vi "MAIN PROGRAM.vi"() -> ()   [LabVIEW 2011]
uses:
  NCML-PhaseSpace/ctrOWLMarker.ctl
  ctlTrialState.ctl
  ctlProtocol.ctl
  ctlProtocolSubID.ctl
  ctlProtocolUnit.ctl
  ctlSeqFNs.ctl
  ctlPkgMain.ctl
  ctlSeqFNs_SubVI PhaseSpace.ctl
  ctlSeqFNs_SubVI ATI.ctl
  ctldistance2plane.ctl
  ctlRecording.ctl
  <vilib>/DAQmx/write.llb/DAQmx Write (Digital 1D U8 1Chan NSamp).vi
  GLOBAL -MAIN.vi
  <vilib>/Utility/file.llb/Write To Spreadsheet File (string).vi
  <vilib>/DAQmx/miscellaneous.llb/DAQmx Fill In Error Info.vi
  <vilib>/Analysis/baseanly.llb/Real Dot Product.vi
  <vilib>/Analysis/NI_AALBase.lvlib
  <vilib>/Utility/VariantDataType/VariantType.lvlib
panel:
  in  "RepeatTrial":bool
  out "Unit Trial count":i32[](array[numeric])
  in  "Recording?":bool=TRUE
  in  "hold criterion (mm)":dbl=250.0 min=0.0 max=500.0 step=1.0
  out "total trials":i32
  in  "Path":path=path "Z:/Yen/NCML-EEGrasp/Data"
  in  "Bias":bool
  out "d (mm)":dbl
  out "ATI":cluster{dbl[][]}[](array[cluster]) {"?" format="%#.2f"}
  out "Current Protocol":T1
  in  "Protocol":T1={"Subject ID"=enum."S000", "1st Handle Left?"=FALSE, "Trial #"=0, "unit"=enum."IL", "unit #"=0, "Trial list"=[], "count in unit"=0, "IL count"=19, "PT count"=3, "postL sessions"=19, "TR max count"=1} {"TR max count" min=1 max=3 step=1; "postL sessions" min=1 max=100 step=1; "PT count" min=1 max=3 step=1}
  out "state":T4
  out "Markers":T5[](array[typedef])
  in  "STOP":bool
  in  "Ready":bool
  out "Date & Time":timestamp format="%<%.3X %x>T"
  # "Main Program"
  # "Recieves data from both SubVIs"
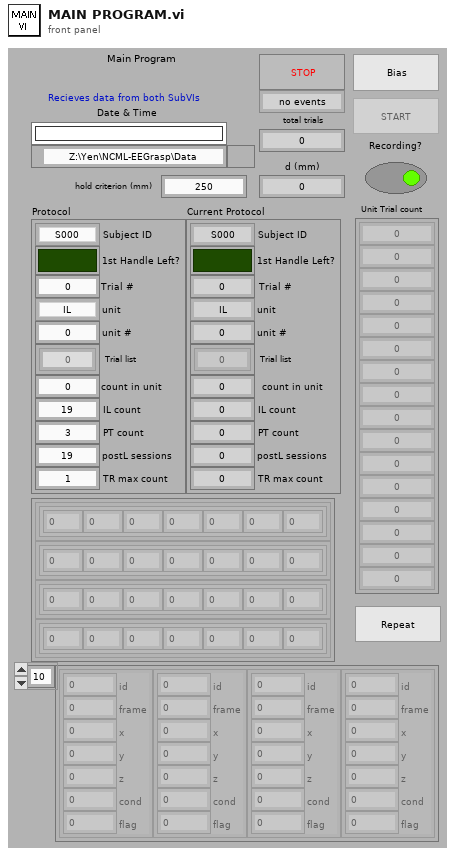
[diagram p1: front panel]
types:
  T1 = typedef "ctlProtocol.ctl" = cluster{"Subject ID":T2, "1st Handle Left?":bool, "Trial #":i32, "unit":T3, "unit #":i32, "Trial list":i32[], "count in unit":i32, "IL count":i32, "PT count":i32, "postL sessions":i32, "TR max count":i32}
  T2 = typedef "ctlProtocolSubID.ctl" = enum16{"S000", "S001", "S002", "S003", "S004", "S005", "S006", "S007"}
  T3 = typedef "ctlProtocolUnit.ctl" = enum16{"IL", "TR", "PT"}
  T4 = typedef "ctlTrialState.ctl" = enum16{"no events", "ready", "start", "hold", "stop", "end"}
  T5 = typedef "ctrOWLMarker.ctl" = cluster{"id":i32, "frame":i32, "x":sgl, "y":sgl, "z":sgl, "cond":sgl, "flag":u32}
  T6 = typedef "ctlPkgMain.ctl" = cluster{"VIRefNm ":refnum<vi>, "PhaseSpace":refnum<queue>, "ATI":refnum<queue>, "Handle Height":dbl, "Results":cluster{"Kc":string, "Cfg":dbl[]}, "CurrPath":path, "state":T4, "tick ini":i64, "Protocol":T1, "PhaseSpace end?":bool, "ATI end?":bool, "trigger task":refnum<k21>, "Markers":T5[], "ATI Data":cluster{dbl[][]}[], "d2plane":T7, "data Path":path, "CurrentProtocol":T1, "tdms data":refnum<k34>, "Recording?":bool}
  T7 = typedef "ctldistance2plane.ctl" = cluster{"1/sqrt(A2+B2+C2)":dbl, "D":dbl, "N":dbl[]}
  T8 = typedef "ctlSeqFNs.ctl" = enum16{"INITIALIZE MAIN", "UpdateProtocol", "UpdatePath", "INITIALIZE Sub", "IDLE", "Bias", "Ready", "RepeatTrial", "Events", "Get PS bias", "Get PhaseSpace", "Get ATI", "Finish", "End PhaseSpace", "End ATI", "ERROR", "EXIT"}
  T9 = enum8{"Enabled", "Disabled", "Disabled and Grayed Out"}
  T10 = typedef "ctlDistance2plane.ctl" = cluster{"1/sqrt(A2+B2+C2)":dbl, "D":dbl, "N":dbl[]}
  T11 = enum16{"ALIGN -CENTER", "ALIGN -TOP LEFT", "ALIGN -AS IS", "ALIGN -CUSTOM"}
  T12 = typedef "ctlSeqFNs_SubVI ATI.ctl" = enum16{"INITIALIZE", "SET HANDLE", "IDLE", "READY", "SEND2MAIN", "CALIB Load", "BIAS", "TRIGGER", "END", "ERROR", "EXIT"}
  T13 = typedef "ctlSeqFNs_SubVI PhaseSpace.ctl" = enum16{"INITIALIZE", "IDLE", "BIAS", "READY", "SEND2MAIN", "LOG2TDMS", "TRIGGER", "END", "ERROR", "EXIT"}
  T14 = enum16{"open", "open or create", "create or replace", "create", "open (read-only)"}
  T15 = typedef "ctlRecording.ctl" = cluster{"recording?":bool, "tdms file":refnum<k34>}
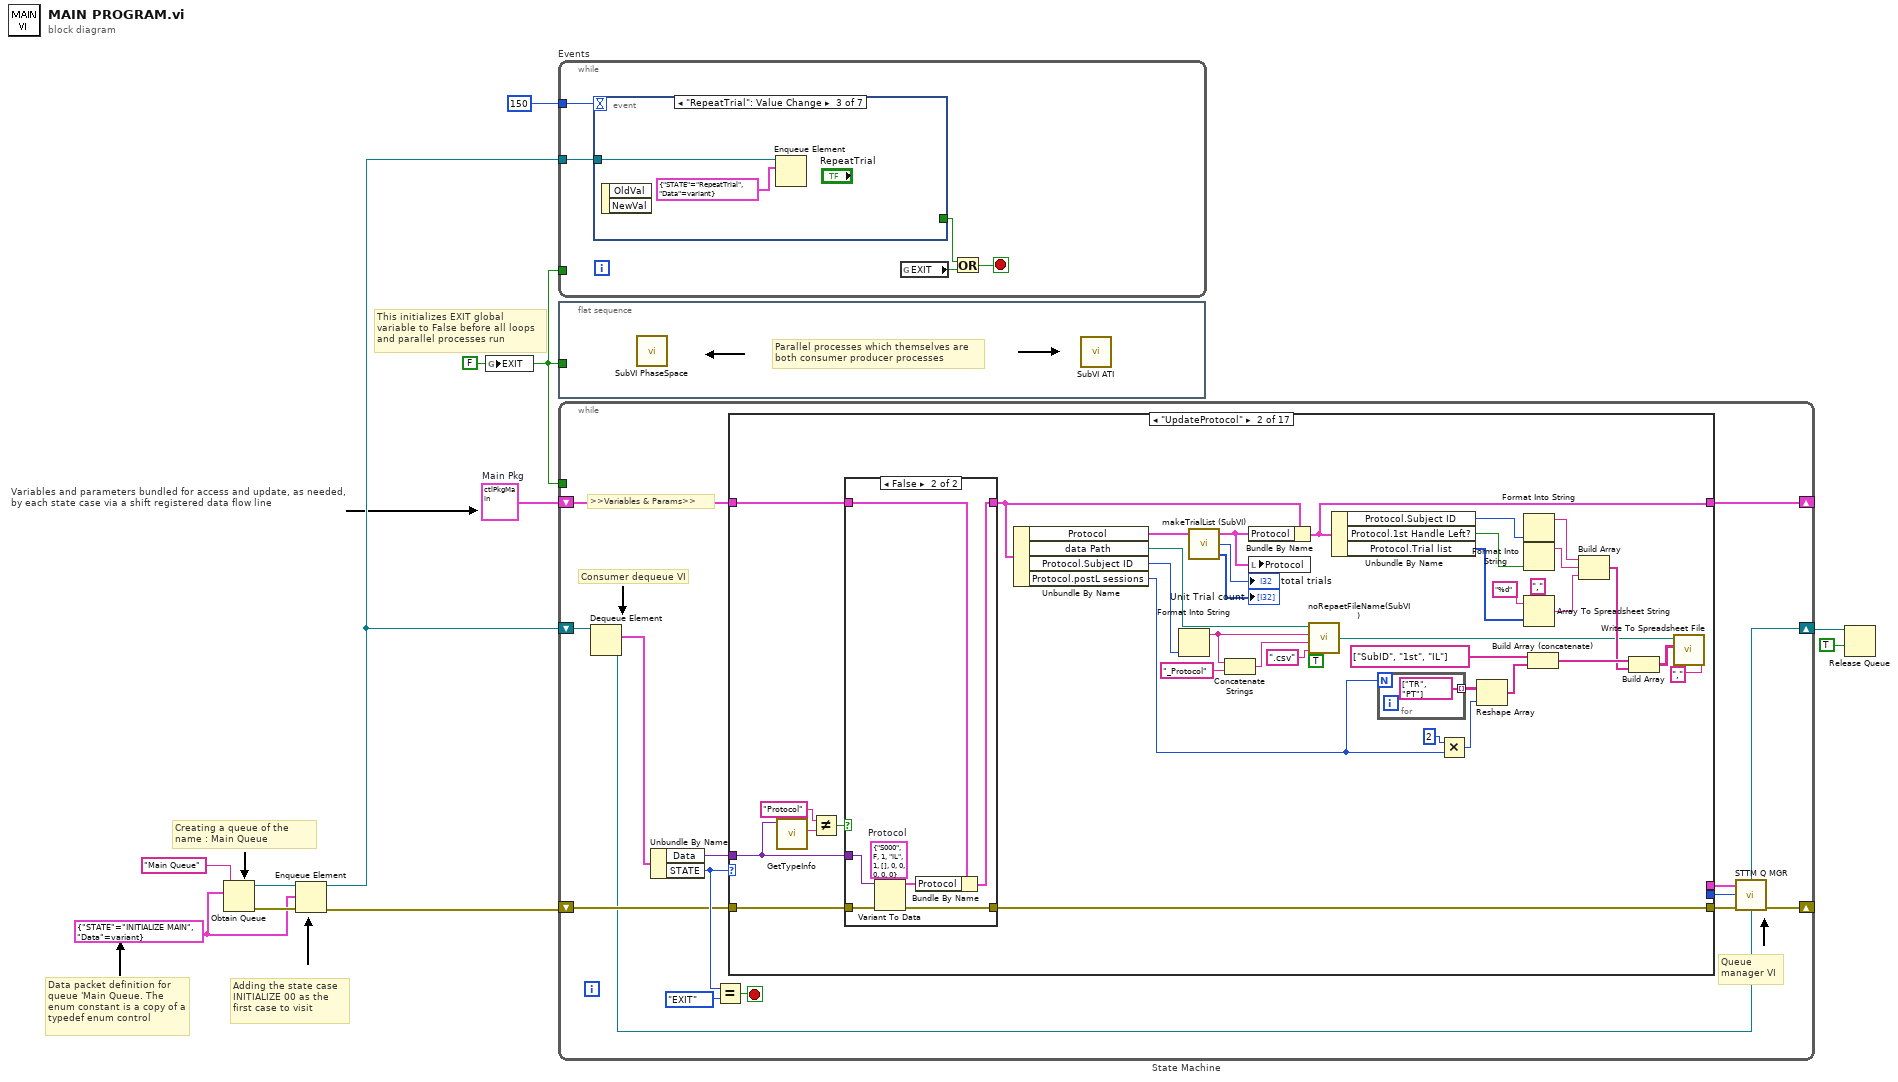
[diagram p0: block diagram]
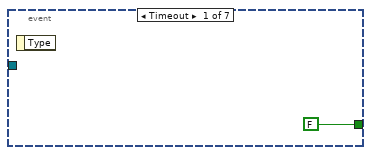
[diagram p2: hidden frame]
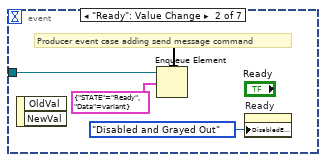
[diagram p3: hidden frame]
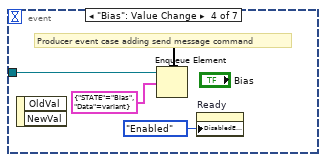
[diagram p4: hidden frame]
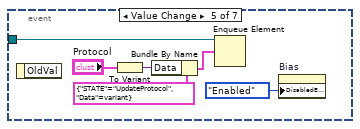
[diagram p5: hidden frame]
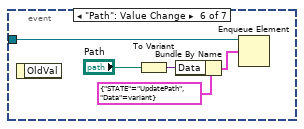
[diagram p6: hidden frame]
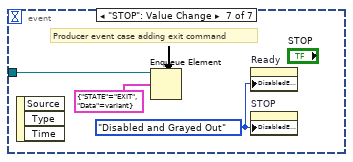
[diagram p7: hidden frame]
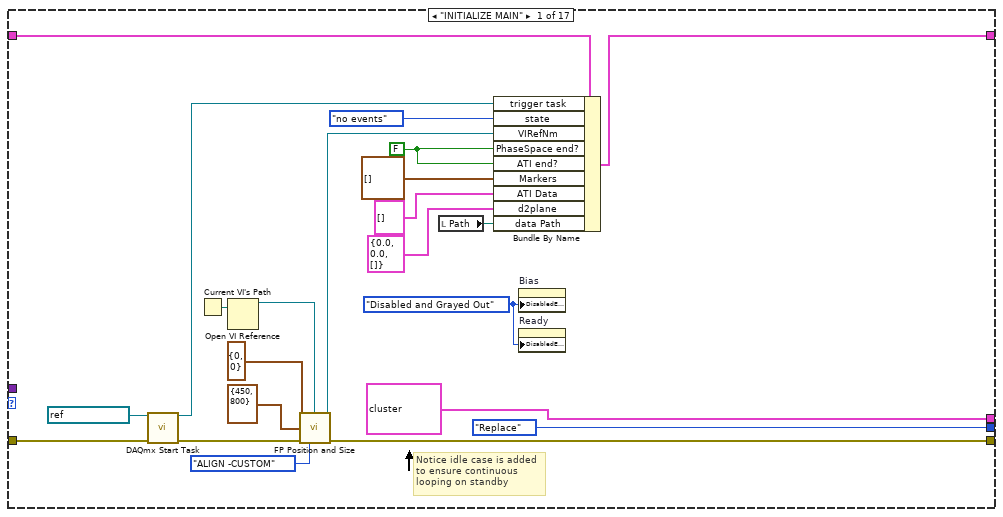
[diagram p8: hidden frame]
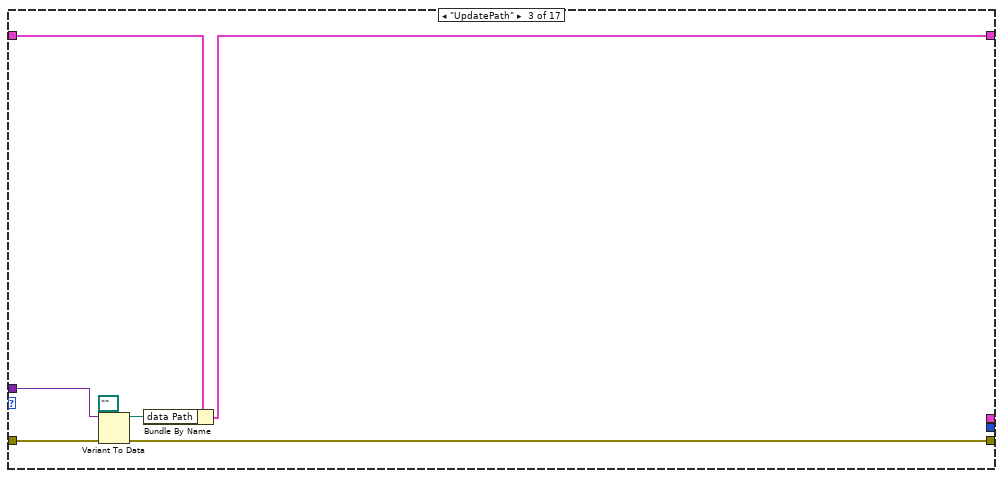
[diagram p10: hidden frame]
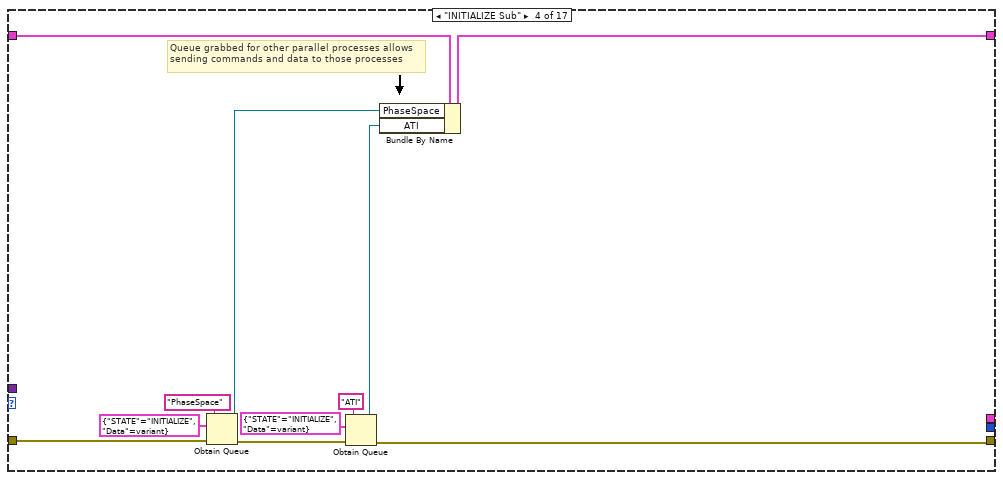
[diagram p11: hidden frame]
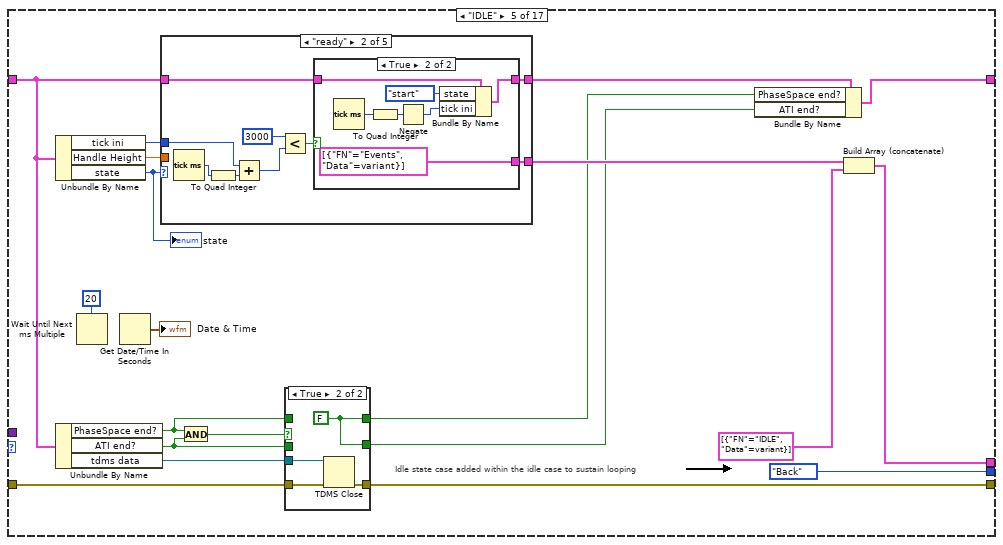
[diagram p12: hidden frame]
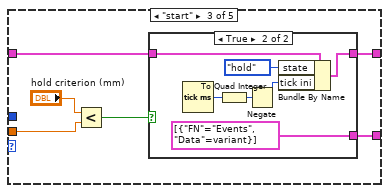
[diagram p16: hidden frame]
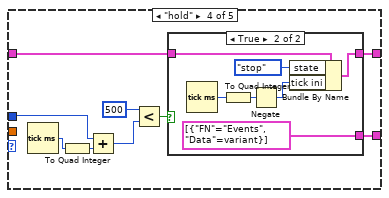
[diagram p18: hidden frame]
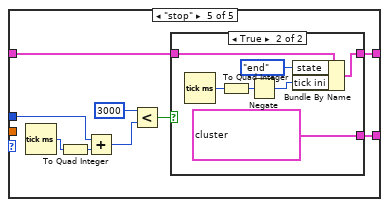
[diagram p20: hidden frame]
diagram:
  w1 = T6 {"VIRefNm "=refnum, "PhaseSpace"=refnum, "ATI"=refnum, "Handle Height"=0.0, "Results"={"Kc"="", "Cfg"=[]}, "CurrPath"=path "", "state"=enum."no events", "tick ini"=0, "Protocol"={"Subject ID"=enum."S000", "1st Handle Left?"=FALSE, "Trial #"=0, "unit"=enum."IL", "unit #"=0, "Trial list"=[], "count in unit"=0, "IL count"=0, "PT count"=0, "postL sessions"=0, "TR max count"=0}, "PhaseSpace end?"=FALSE, "ATI end?"=FALSE, "trigger task"="", "Markers"=[], "ATI Data"=[], "d2plane"={"1/sqrt(A2+B2+C2)"=0.0, "D"=0.0, "N"=[]}, "data Path"=path "", "CurrentProtocol"={"Subject ID"=enum."S000", "1st Handle Left?"=FALSE, "Trial #"=0, "unit"=enum."IL", "unit #"=0, "Trial list"=[], "count in unit"=0, "IL count"=0, "PT count"=0, "postL sessions"=0, "TR max count"=0}, "tdms data"=refnum, "Recording?"=FALSE}  # Main Pkg
  w4 = FALSE
  w5 = cluster{"STATE":T8, "Data":variant} {"STATE"=enum."INITIALIZE MAIN", "Data"=variant} ("element")
  # "This initializes EXIT global variable to False before all loops and parallel processes run"
  # "Data packet definition for queue 'Main Queue. The enum constant is a copy of a typedef enum control"
  # "Adding the state case INITIALIZE 00 as the first case to visit"
  # "Creating a queue of the name : Main Queue"
  # "Variables and parameters bundled for access and update, as needed,  by each state case via a shift registered data flow line"
  n1 = Obtain Queue(name (unnamed)="Main Queue" ("Queue Name"), element data type=w5) -> (queue out=w3:refnum<queue>, error out=w7:errorcluster)  [unwired: 3 in, 1 out]
  n2 = Enqueue Element(queue=w3, element=w5, error in (no error)=w7) -> (queue out=w2:refnum<queue>, error out=w6:errorcluster)  [unwired: 1 in, 1 out]
  n3 = global write "GLOBAL -MAIN.vi" "EXIT"(w4) -> ()
  n4 = while "Events" {
    tunnel: 150 -> [w16]
    tunnel: w4 -> [_]
    tunnel: w2 -> [w12]
    stop <- w13 stop-if-true
    n5 = event shown="[2] \"RepeatTrial\": Value Change" {
      selector: _ -> [_ _ _ _ _ _ _]
      dyn-events: _ -> [_ _ _ _ _ _ _]
      timeout: w16 -> [_ _ _ _ _ _ _]
      tunnel: [FALSE _ _ _ _ _ _] -> w15
      tunnel: w12 -> [_ w20 w22 w25 w30 w35 w39]
      event Timeout {
        n6 = event-data() -> ()  [unwired: 1 in, 1 out]
      }
      event "Ready": Value Change {
        # "Producer event case adding send message command"
        n7 = event-data() -> ()  [unwired: 1 in, 2 out]
        n8 = Enqueue Element(queue=w20, element=cluster{"STATE":T8, "Data":variant} {"STATE"=enum."Ready", "Data"=variant}) -> ()  [unwired: 2 in, 3 out]
        n9 = property on="Ready" class="Bool"("DisabledEnum"=T9."Disabled and Grayed Out" ("Disabled")) -> ()  [unwired: 2 in, 2 out]
      }
      event "RepeatTrial": Value Change {
        n10 = event-data() -> ()  [unwired: 1 in, 2 out]
        n11 = Enqueue Element(queue=w22, element=cluster{"STATE":T8, "Data":variant} {"STATE"=enum."RepeatTrial", "Data"=variant}) -> ()  [unwired: 2 in, 3 out]
      }
      event "Bias": Value Change {
        # "Producer event case adding send message command"
        n12 = event-data() -> ()  [unwired: 1 in, 2 out]
        n13 = Enqueue Element(queue=w25, element=cluster{"STATE":T8, "Data":variant} {"STATE"=enum."Bias", "Data"=variant}) -> ()  [unwired: 2 in, 3 out]
        n14 = property on="Ready" class="Bool"("DisabledEnum"=T9."Enabled" ("Disabled")) -> ()  [unwired: 2 in, 2 out]
      }
      event Value Change {
        n15 = event-data() -> ()  [unwired: 1 in, 1 out]
        n16 = To Variant(anything="Protocol") -> (Variant=w28:variant)
        n17 = Bundle By Name(cluster=cluster{"STATE":T8, "Data":variant} {"STATE"=enum."UpdateProtocol", "Data"=variant} ("element"), "Data"=w28) -> (w29:cluster{"STATE":T8, "Data":variant})
        n18 = Enqueue Element(queue=w30, element=w29) -> ()  [unwired: 2 in, 3 out]
        n19 = property on="Bias" class="Bool"("DisabledEnum"=T9."Enabled" ("Disabled")) -> ()  [unwired: 2 in, 2 out]
      }
      event "Path": Value Change {
        n20 = event-data() -> ()  [unwired: 1 in, 1 out]
        n21 = To Variant(anything="Path") -> (Variant=w33:variant)
        n22 = Bundle By Name(cluster=cluster{"STATE":T8, "Data":variant} {"STATE"=enum."UpdatePath", "Data"=variant} ("element"), "Data"=w33) -> (w34:cluster{"STATE":T8, "Data":variant})
        n23 = Enqueue Element(queue=w35, element=w34) -> ()  [unwired: 2 in, 3 out]
      }
      event "STOP": Value Change {
        w37 = T9."Disabled and Grayed Out" ("Disabled")
        # "Producer event case adding exit command"
        n24 = event-data() -> ()  [unwired: 1 in, 3 out]
        n25 = Enqueue Element(queue=w39, element=cluster{"STATE":T8, "Data":variant} {"STATE"=enum."EXIT", "Data"=variant}) -> ()  [unwired: 2 in, 3 out]
        n26 = property on="Ready" class="Bool"("DisabledEnum"=w37) -> ()  [unwired: 2 in, 2 out]
        n27 = property on="STOP" class="Bool"("DisabledEnum"=w37) -> ()  [unwired: 2 in, 2 out]
      }
    }
    n28 = global read "GLOBAL -MAIN.vi" "EXIT"() -> (w14:bool)
    n29 = Or(x=w15, y=w14) -> (x .or. y?=w13:bool)
  }
  n30 = flat-sequence {
    tunnel: w4 -> [_]
    frame #0 {
      # "Parallel processes which themselves are both consumer producer processes"
      n31 = call "SubVI PhaseSpace.vi"() -> ()  [unwired: 16 in]
      n32 = call "SubVI ATI.vi"() -> ()  [unwired: 16 in]
    }
  }
  n33 = while "State Machine" {
    shift-right: [w47] -> _
    shift-left: w6 -> [w46]
    shift-right: [w40] -> w9
    shift-left: w2 -> [w53]
    tunnel: w4 -> [_]
    shift-right: [w43] -> _
    shift-left: w1 -> [w44]
    stop <- w45 stop-if-true
    # "Queue manager VI"
    # "Consumer dequeue VI"
    # ">>Variables & Params>>"
    n34 = Dequeue Element(queue=w53) -> (queue out=w40:refnum<queue>, element=w52:cluster{"STATE":T8, "Data":variant})  [unwired: 2 in, 2 out]
    n35 = Unbundle By Name(w52) -> ("Data"=w51:variant, "STATE"=w50:T8)
    n36 = Equal?(x=w50, y=ctlSeqFNs."EXIT" ("FN")) -> (x = y?=w45:bool)
    n37 = case shown="\"UpdateProtocol\"" w50 {
      tunnel: w46 -> [w60 w112 w128 w132 w151 w243 w277 w287 w305 w363 w371 w378 w398 w400 w404 w408 w411]
      tunnel: [w70 w113 w129 w133 w150 w241 w274 w287 w300 w362 w370 w377 w391 w400 w404 w407 w414] -> w48
      tunnel: w51 -> [_ w111 w127 _ _ _ _ _ _ w365 w372 w379 _ _ _ _ _]
      tunnel: [cluster{"FN":T8, "Data":variant}[] [{"FN"=enum."INITIALIZE Sub", "Data"=variant}, {"FN"=enum."IDLE", "Data"=variant}] _ _ _ w157 _ cluster{"FN":T8, "Data":variant}[] [{"FN"=enum."Events", "Data"=variant}] _ _ _ _ _ _ _ _ _ _] -> w41
      tunnel: w44 -> [w64 w114 w131 w142 w152 w237 w259 w285 w314 w349 w369 w375 w380 w402 w406 w409 w420]
      tunnel: [w69 w86 w130 w141 w148 w237 w275 w286 w314 w361 w368 w374 w381 w401 w405 w409 w420] -> w43
      tunnel: [enum16{"Back", "Front", "Replace"}."Replace" ("FNs") _ _ _ enum16{"Back", "Front", "Replace"}."Back" ("FNs") _ enum16{"Back", "Front", "Replace"}."Front" ("FNs") _ _ _ _ _ _ _ _ _ _] -> w42
      frame "INITIALIZE MAIN" {
        w54 = T9."Disabled and Grayed Out" ("Disabled")
        w63 = FALSE ("PhaseSpace end?")
        # "Notice idle case is added to ensure continuous looping on standby"
        n38 = call <vilib>:"DAQmx Start Task.vi"("task/channels in"=refnum<k21> "TriggerPort" ("DAQmx Task Name"), "error in"=w60) -> ("task out"=w61:refnum<k21>, "error out"=w59:errorcluster)  [unwired: 12 in]
        n39 = Current VI's Path() -> (path=w71:path)
        n40 = Open VI Reference(vi path=w71) -> (vi reference=w72:refnum<vi>)  [unwired: 5 in, 1 out]
        n41 = call "FP Position and Size.vi"("VIRefNum  IN"=w72, "Poistion"=cluster{"left":i16, "top":i16} {"left"=0, "top"=0}, "Size"=cluster{"right":i16, "bottom":i16} {"right"=450, "bottom"=800}, "error in (no error)"=w59, "Mode"=T11."ALIGN -CUSTOM") -> ("VIRefNum OUT"=w68:refnum<vi>, "error out"=w70:errorcluster)  [unwired: 9 in]
        n42 = local read "Path"() -> (w55:path)
        n43 = Bundle By Name(cluster=w64, "trigger task"=w61, "state"=ctlTrialState."no events", "VIRefNm"=w68, "PhaseSpace end?"=w63, "ATI end?"=w63, "Markers"=T5[] [], "ATI Data"=cluster{dbl[][]}[] [] ("Data"), "d2plane"=T10 {"1/sqrt(A2+B2+C2)"=0.0, "D"=0.0, "N"=[]}, "data Path"=w55) -> (w69:T6)
        n44 = property on="Bias" class="Bool"("DisabledEnum"=w54) -> ()  [unwired: 2 in, 2 out]
        n45 = property on="Ready" class="Bool"("DisabledEnum"=w54) -> ()  [unwired: 2 in, 2 out]
      }
      frame "UpdateProtocol" {
        n46 = call <vilib>:"GetTypeInfo.vi"("Variant"=w111) -> ("Name"=w110:string)  [unwired: 6 in, 4 out]
        n47 = Not Equal?(x="Protocol", y=w110) -> (x != y?=w108:bool)
        n48 = case shown="False" w108 {
          tunnel: w114 -> [w117 w124]
          tunnel: [w117 w123] -> w88
          tunnel: [w116 w118] -> w113
          tunnel: w112 -> [w116 w120]
          tunnel: w111 -> [_ w119]
          frame True {
          }
          frame False {
            w122 = T1 {"Subject ID"=enum."S000", "1st Handle Left?"=FALSE, "Trial #"=1, "unit"=enum."IL", "unit #"=1, "Trial list"=[], "count in unit"=0, "IL count"=0, "PT count"=0, "postL sessions"=0, "TR max count"=0}  # Protocol
            n49 = Variant To Data(error in=w120, type=w122, Variant=w119) -> (data=w121:T1, error out=w118:errorcluster)
            n50 = Bundle By Name(cluster=w124, "Protocol"=w121) -> (w123:T6)
          }
        }
        n51 = Unbundle By Name(w88) -> ("Protocol"=w89:T1, "data Path"=w81:path, "Protocol.Subject ID"=w82:T2, "Protocol.postL sessions"=w83:i32)
        n52 = Format Into String(w82) -> (resulting string=w80:string)  [unwired: 3 in, 1 out]
        n53 = call "makeTrialList (SubVI).vi"("Protocol in"=w89) -> ("Unit Trial count"=→"Unit Trial count":i32[], "total trial count"=→"total trials":i32, "Protocol out"=w87:T1)  [unwired: 2 in]
        n54 = Concatenate Strings(w80, "_Protocol") -> (w79:string)
        n55 = Bundle By Name(cluster=w88, "Protocol"=w87) -> (w86:T6)
        n56 = local write "Protocol"(w87) -> ()
        n57 = call "noRepaetFileName(SubVI).vi"("prompt overwrite?"=TRUE, "ext"=".csv" ("string"), "file name"=w79, "subID"=w80, "directory Path"=w81) -> ("file path out"=w76:path)  [unwired: 1 in]
        n58 = Unbundle By Name(w86) -> ("Protocol.Subject ID"=w100:T2, "Protocol.1st Handle Left?"=w99:bool, "Protocol.Trial list"=w96:i32[])
        n59 = for {
          N: w83 -> [_]
          tunnel: [string[] ["TR", "PT"]] -> w106 mode=indexing
        }
        n60 = Multiply(x=2 ("y"), y=w83) -> (x*y=w105:i32)
        n61 = Reshape Array(w106, w105) -> (w104:string[])
        n62 = Format Into String(w100) -> (resulting string=w98:string)  [unwired: 3 in, 1 out]
        n63 = Format Into String(w99) -> (resulting string=w97:string)  [unwired: 3 in, 1 out]
        n64 = Array To Spreadsheet String(delimiter (Tab)=",", array=w96, 3:"%d" ("format string")) -> (spreadsheet string=w94:string)
        n65 = Build Array (concatenate)(string[] ["SubID", "1st", "IL"], w104) -> (w102:string[])
        n66 = Build Array(w98, w97, w94) -> (w92:string[])
        n67 = Build Array(w102, w92) -> (w93:string[][])
        n68 = call-poly <vilib>:"Write To Spreadsheet File.vi"("delimiter (\\t)"="," ("delimiter (\\t)"), "2D data"=w93, "file path (dialog if empty)"=w76) -> ()  [unwired: 5 in, 1 out]
      }
      frame "UpdatePath" {
        n69 = Variant To Data(error in=w128, type=path "", Variant=w127) -> (data=w126:path, error out=w129:errorcluster)
        n70 = Bundle By Name(cluster=w131, "data Path"=w126) -> (w130:T6)
      }
      frame "INITIALIZE Sub" {
        # "Queue grabbed for other parallel processes allows sending commands and data to those processes"
        n71 = Obtain Queue(name (unnamed)="PhaseSpace", element data type=cluster{"STATE":T13, "Data":variant} {"STATE"=enum."INITIALIZE", "Data"=variant} ("element"), error in (no error)=w132) -> (queue out=w135:refnum<queue>, error out=w140:errorcluster)  [unwired: 2 in, 1 out]
        n72 = Obtain Queue(name (unnamed)="ATI", element data type=cluster{"STATE":T12, "Data":variant} {"STATE"=enum."INITIALIZE", "Data"=variant} ("element"), error in (no error)=w140) -> (queue out=w134:refnum<queue>, error out=w133:errorcluster)  [unwired: 2 in, 1 out]
        n73 = Bundle By Name(cluster=w142, "PhaseSpace"=w135, "ATI"=w134) -> (w141:T6)
      }
      frame "IDLE" {
        # "Idle state case added within the idle case to sustain looping"
        n74 = Unbundle By Name(w152) -> ("tick ini"=w154:i64, "Handle Height"=w159:dbl, "state"=w160:T4)
        "state" <- w160
        n75 = Unbundle By Name(w152) -> ("PhaseSpace end?"=w144:bool, "ATI end?"=w147:bool, "tdms data"=w153:refnum<k34>)
        n76 = Wait Until Next ms Multiple(millisecond multiple=u32 20) -> ()  [unwired: 1 out]
        n77 = Get Date/Time In Seconds() -> (seconds since 1Jan1904=→"Date & Time":timestamp)
        n78 = case shown="\"ready\"" w160 {
          tunnel: w159 -> [_ _ w189 _ _]
          tunnel: w152 -> [w170 w179 w193 w210 w227]
          tunnel: [w170 w178 w192 w209 w226] -> w149
          tunnel: [_ w177 w188 w208 w225] -> w155
          tunnel: w154 -> [_ w175 _ w203 w220]
          frame "no events", Default {
          }
          frame "ready" {
            n79 = Tick Count (ms)() -> (millisecond timer value=w176:u32)
            n80 = To Quad Integer(1:w176) -> (0:w174:i64)
            n81 = Add(x=w175, y=w174) -> (x+y=w172:i64)
            n82 = Less?(x=i64 3000 ("Time Target (s)"), y=w172) -> (x < y?=w173:bool)
            n83 = case shown="True" w173 {
              tunnel: w179 -> [w180 w187]
              tunnel: [w180 w186] -> w178
              tunnel: [_ cluster{"FN":T8, "Data":variant}[] [{"FN"=enum."Events", "Data"=variant}]] -> w177
              frame False {
              }
              frame True {
                n84 = Tick Count (ms)() -> (millisecond timer value=w182:u32)
                n85 = To Quad Integer(1:w182) -> (0:w183:i64)
                n86 = Negate(x=w183) -> (-x=w181:i64)
                n87 = Bundle By Name(cluster=w187, "state"=ctlTrialState."start", "tick ini"=w181) -> (w186:T6)
              }
            }
          }
          frame "start" {
            n88 = Less?(x="hold criterion (mm)", y=w189) -> (x < y?=w191:bool)
            n89 = case shown="True" w191 {
              tunnel: w193 -> [w194 w201]
              tunnel: [w194 w200] -> w192
              tunnel: [_ cluster{"FN":T8, "Data":variant}[] [{"FN"=enum."Events", "Data"=variant}]] -> w188
              frame False {
              }
              frame True {
                n90 = Tick Count (ms)() -> (millisecond timer value=w197:u32)
                n91 = To Quad Integer(1:w197) -> (0:w196:i64)
                n92 = Negate(x=w196) -> (-x=w195:i64)
                n93 = Bundle By Name(cluster=w201, "state"=ctlTrialState."hold", "tick ini"=w195) -> (w200:T6)
              }
            }
          }
          frame "hold" {
            n94 = Tick Count (ms)() -> (millisecond timer value=w207:u32)
            n95 = To Quad Integer(1:w207) -> (0:w206:i64)
            n96 = Add(x=w203, y=w206) -> (x+y=w205:i64)
            n97 = Less?(x=i64 500 ("Time Target (s)"), y=w205) -> (x < y?=w202:bool)
            n98 = case shown="True" w202 {
              tunnel: w210 -> [w211 w218]
              tunnel: [w211 w217] -> w209
              tunnel: [_ cluster{"FN":T8, "Data":variant}[] [{"FN"=enum."Events", "Data"=variant}]] -> w208
              frame False {
              }
              frame True {
                n99 = Tick Count (ms)() -> (millisecond timer value=w214:u32)
                n100 = To Quad Integer(1:w214) -> (0:w213:i64)
                n101 = Negate(x=w213) -> (-x=w212:i64)
                n102 = Bundle By Name(cluster=w218, "state"=ctlTrialState."stop", "tick ini"=w212) -> (w217:T6)
              }
            }
          }
          frame "stop" {
            n103 = Tick Count (ms)() -> (millisecond timer value=w224:u32)
            n104 = To Quad Integer(1:w224) -> (0:w223:i64)
            n105 = Add(x=w220, y=w223) -> (x+y=w222:i64)
            n106 = Less?(x=i64 3000 ("Time Target (s)"), y=w222) -> (x < y?=w219:bool)
            n107 = case shown="True" w219 {
              tunnel: w227 -> [w228 w235]
              tunnel: [w228 w234] -> w226
              tunnel: [_ cluster{"FN":T8, "Data":variant}[] [{"FN"=enum."Events", "Data"=variant}, {"FN"=enum."Finish", "Data"=variant}]] -> w225
              frame False {
              }
              frame True {
                n108 = Tick Count (ms)() -> (millisecond timer value=w230:u32)
                n109 = To Quad Integer(1:w230) -> (0:w231:i64)
                n110 = Negate(x=w231) -> (-x=w229:i64)
                n111 = Bundle By Name(cluster=w235, "state"=ctlTrialState."end", "tick ini"=w229) -> (w234:T6)
              }
            }
          }
        }
        n112 = And(x=w144, y=w147) -> (x .and. y?=w143:bool)
        n113 = case shown="True" w143 {
          tunnel: w153 -> [_ w169]
          tunnel: w151 -> [w165 w168]
          tunnel: [w165 w167] -> w150
          tunnel: [w164 w166] -> w146
          tunnel: w144 -> [w164 _]
          tunnel: [w163 w166] -> w145
          tunnel: w147 -> [w163 _]
          frame False {
          }
          frame True {
            w166 = FALSE
            n114 = TDMS Close(8:w168, 11:w169) -> (0:w167:errorcluster)  [unwired: 1 out]
          }
        }
        n115 = Bundle By Name(cluster=w149, "PhaseSpace end?"=w146, "ATI end?"=w145) -> (w148:T6)
        n116 = Build Array (concatenate)(w155, cluster{"FN":T8, "Data":variant}[] [{"FN"=enum."IDLE", "Data"=variant}]) -> (w157:cluster{"FN":T8, "Data":variant}[])
      }
      frame "Bias" {
        n117 = Unbundle By Name(w237) -> ("PhaseSpace"=w239:refnum<queue>, "ATI"=w240:refnum<queue>)
        n118 = Enqueue Element(queue=w240, element=cluster{"STATE":T12, "Data":variant} {"STATE"=enum."BIAS", "Data"=variant}, error in (no error)=w243) -> (error out=w242:errorcluster)  [unwired: 1 in, 2 out]
        n119 = Enqueue Element(queue=w239, element=cluster{"STATE":T13, "Data":variant} {"STATE"=enum."BIAS", "Data"=variant}, error in (no error)=w242) -> (error out=w241:errorcluster)  [unwired: 1 in, 2 out]
      }
      frame "Ready" {
        n120 = Unbundle By Name(w259) -> ("Protocol"=w245:T1, "data Path"=w256:path, "PhaseSpace"=w263:refnum<queue>, "ATI"=w264:refnum<queue>)
        n121 = in-place {
          n122 = in-place-cluster #1(w245) -> ("Trial #"=w280:i32, "unit #"=w283:i32, "count in unit"=w282:i32)
          n123 = Increment(x=w280) -> (x+1=w278:i32)
          n124 = Increment(x=w282) -> (x+1=w279:i32)
          n125 = Increment(x=w283) -> (x+1=w281:i32)
          n126 = in-place-cluster #1("Trial #"=w278, "unit #"=w281, "count in unit"=w279) -> (→"Current Protocol":T1)
        }
        n127 = call "updateTrialInfo (SubVI).vi"("data Path"=w256, "pre Protocol"=w245) -> ("file path out"=w252:path, "next"=w246:T1)
        n128 = Strip Path(path=w252) -> (stripped path=w251:path)  [unwired: 1 out]
        n129 = Build Path(base path=w251, name or relative path="dummy") -> (appended path=w249:path)
        n130 = Select(t=w252, s="Recording?", f=w249) -> (s? t:f=w253:path)
        n131 = TDMS Open(6:FALSE ("disable buffering? (T)"), 10:T14."create or replace" ("operation"), 11:w253) -> (3:w248:refnum<k34>)  [unwired: 3 in, 1 out]
        n132 = Bundle By Name(cluster=T15 {"recording?"=FALSE, "tdms file"=refnum} ("output cluster"), "tdms file"=w248, "recording?"="Recording?") -> (w257:T15)
        n133 = Tick Count (ms)() -> (millisecond timer value=w267:u32)
        n134 = To Quad Integer(1:w267) -> (0:w266:i64)
        n135 = To Variant(anything=w257) -> (Variant=w262:variant)
        n136 = Negate(x=w266) -> (-x=w265:i64)
        n137 = Bundle By Name(cluster=cluster{"STATE":T12, "Data":variant} {"STATE"=enum."READY", "Data"=variant} ("element"), "Data"=w262) -> (w260:cluster{"STATE":T12, "Data":variant})
        n138 = Bundle By Name(cluster=w259, "CurrentProtocol"=w245, "Protocol"=w246, "state"=ctlTrialState."ready", "tick ini"=w265, "tdms data"=w248, "Recording?"="Recording?") -> (w275:T6)
        n139 = Enqueue Element(queue=w264, element=w260, error in (no error)=w277) -> (error out=w276:errorcluster)  [unwired: 1 in, 2 out]
        n140 = To Variant(anything=w257) -> (Variant=w268:variant)
        n141 = Bundle By Name(cluster=cluster{"STATE":T13, "Data":variant} {"STATE"=enum."READY", "Data"=variant} ("element"), "Data"=w268) -> (w269:cluster{"STATE":T13, "Data":variant})
        n142 = Enqueue Element(queue=w263, element=w269, error in (no error)=w276) -> (error out=w274:errorcluster)  [unwired: 1 in, 2 out]
      }
      frame "RepeatTrial" {
        n143 = Unbundle By Name(w285) -> ("CurrentProtocol"=w284:T1)
        n144 = Bundle By Name(cluster=w285, "Protocol"=w284) -> (w286:T6)
      }
      frame "Events" {
        n145 = Unbundle By Name(w314) -> ("PhaseSpace"=w291:refnum<queue>, "ATI"=w290:refnum<queue>, "CurrentProtocol.unit"=w288:T3, "CurrentProtocol.1st Handle Left?"=w289:bool, "state"=w308:T4, "trigger task"=w307:refnum<k21>)
        n146 = case shown="\"start\"" w308 {
          selector: w308 -> [w321 w324 w335 w338 w341 w344]
          tunnel: [w321 w324 w335 w338 w341 w344] -> w313
          tunnel: [u8 0 ("element") u8 9 ("element") u8 17 ("element") u8 33 ("element") u8 65 ("element") u8 129 ("element")] -> w310
          tunnel: ["Finish" ("name or relative path") "Ready" ("name or relative path") w326 "Hold" ("name or relative path") "Relax" ("name or relative path") "Finish" ("name or relative path")] -> w295
          tunnel: w289 -> [_ _ w325 _ _ _]
          tunnel: w288 -> [_ _ w328 _ _ _]
          frame "no events", Default {
          }
          frame "ready" {
          }
          frame "start" {
            n147 = Not Equal?(x=w328, y=ctlProtocolUnit."TR" ("Protocol.unit")) -> (x != y?=w329:bool)
            n148 = Not(x=w325) -> (.not. x?=w330:bool)
            n149 = Select(t=w325, s=w329, f=w330) -> (s? t:f=w332:bool)
            n150 = Select(t="Left" ("name or relative path"), s=w332, f="RIght") -> (s? t:f=w326:string)
          }
          frame "hold" {
          }
          frame "stop" {
          }
          frame "end" {
          }
        }
        n151 = To Variant(anything=w313) -> (Variant=w312:variant)
        n152 = Build Array(w310, u8 0 ("element")) -> (w311:u8[])
        n153 = Bundle By Name(cluster=cluster{"STATE":T12, "Data":variant} {"STATE"=enum."TRIGGER", "Data"=variant} ("element"), "Data"=w312) -> (w315:cluster{"STATE":T12, "Data":variant})
        n154 = Enqueue Element(queue=w290, element=w315, error in (no error)=w305) -> (error out=w306:errorcluster)  [unwired: 1 in, 2 out]
        n155 = call-poly <vilib>:"DAQmx Write.vi"("task/channels in"=w307, "data"=w311, "error in"=w305) -> ("error out"=w303:errorcluster)  [unwired: 10 in, 2 out]
        n156 = Bundle By Name(cluster=cluster{"STATE":T13, "Data":variant} {"STATE"=enum."TRIGGER", "Data"=variant} ("element"), "Data"=w312) -> (w316:cluster{"STATE":T13, "Data":variant})
        n157 = Enqueue Element(queue=w291, element=w316, error in (no error)=w305) -> (error out=w304:errorcluster)  [unwired: 1 in, 2 out]
        n158 = call <vilib>:"Application Directory.vi"() -> ("Application Directory"=w297:path)
        n159 = Merge Errors(w304, w306, w303) -> (w299:errorcluster)
        n160 = Build Path(base path=w297, name or relative path="audio cues") -> (appended path=w294:path)
        n161 = Concatenate Strings(w295, ".wav" ("name or relative path")) -> (w293:string)
        n162 = Build Path(base path=w294, name or relative path=w293) -> (appended path=w292:path)
        n163 = call <vilib>:"Sound File Read Simple.vi"("error in (no error)"=w299, "path"=w292) -> ("error out"=w301:errorcluster, "data"=w302:waveform(dbl)[])  [unwired: 6 in, 2 out]
        n164 = call "Play Waveform"("Data"=w302, "error in"=w301) -> ("error out"=w300:errorcluster)  [unwired: 17 in]
      }
      frame "Get PhaseSpace" {
        n165 = Variant To Data(error in=w363, type=T5[] [] ("Markers"), Variant=w365) -> (data=w348:T5[], error out=w362:errorcluster)
        "Markers" <- w348
        n166 = Unbundle By Name(w349) -> ("d2plane.1/sqrt(A2+B2+C2)"=w347:dbl, "d2plane.D"=w346:dbl, "d2plane.N"=w345:dbl[])
        n167 = Reverse 1D Array(array=w348) -> (reversed array=w360:T5[])
        n168 = Index Array(array=w360) -> (element #4=w359:T5)  [unwired: 4 in, 3 out]
        n169 = Unbundle By Name(w359) -> ("x"=w358:sgl, "y"=w357:sgl, "z"=w356:sgl)
        n170 = Build Array(w358, w357, w356) -> (w355:sgl[])
        n171 = To Double Precision Float(number=w355) -> (double precision float=w354:dbl[])
        n172 = call-poly <vilib>:"Dot Product.vi"("Y Vector"=w354, "X Vector"=w345) -> ("X * Y"=w353:dbl)  [unwired: 1 out]
        n173 = Add(x=w346, y=w353) -> (x+y=w352:dbl)
        n174 = Absolute Value(x=w352) -> (abs(x)=w351:dbl)
        n175 = Multiply(x=w347, y=w351) -> (x*y=w350:dbl)
        "d (mm)" <- w350
        n176 = Bundle By Name(cluster=w349, "Handle Height"=w350, "Markers"=w348) -> (w361:T6)
      }
      frame "Get PS bias" {
        n177 = Variant To Data(error in=w371, type=T7 {"1/sqrt(A2+B2+C2)"=0.0, "D"=0.0, "N"=[]}, Variant=w372) -> (data=w367:T7, error out=w370:errorcluster)
        n178 = Bundle By Name(cluster=w369, "d2plane"=w367) -> (w368:T6)
      }
      frame "Get ATI" {
        n179 = Variant To Data(error in=w378, type=cluster{dbl[][]}[] [] ("Data"), Variant=w379) -> (data=w373:cluster{dbl[][]}[], error out=w377:errorcluster)
        "ATI" <- w373
        n180 = Bundle By Name(cluster=w375, "ATI Data"=w373) -> (w374:T6)
      }
      frame "Finish" {
        n181 = Unbundle By Name(w380) -> ("Protocol.Trial list"=w388:i32[], "Protocol.Trial #"=w386:i32, "PhaseSpace"=w396:refnum<queue>, "ATI"=w395:refnum<queue>)
        n182 = Add Array Elements(numeric array=w388) -> (sum=w387:i32)
        n183 = Enqueue Element(queue=w395, element=cluster{"STATE":T12, "Data":variant} {"STATE"=enum."END", "Data"=variant}, error in (no error)=w398) -> (error out=w397:errorcluster)  [unwired: 1 in, 2 out]
        n184 = Bundle By Name(cluster=w380, "state"=ctlTrialState."no events", "Markers"=T5[] [], "ATI Data"=cluster{dbl[][]}[] [] ("Data")) -> (w381:T6)
        n185 = Greater?(x=w387, y=w386) -> (0:w385:bool)
        n186 = Enqueue Element(queue=w396, element=cluster{"STATE":T13, "Data":variant} {"STATE"=enum."END", "Data"=variant}, error in (no error)=w397) -> (error out=w391:errorcluster)  [unwired: 1 in, 2 out]
        n187 = Select(t=T9."Enabled" ("Disabled"), s=w385, f=T9."Disabled and Grayed Out" ("Disabled")) -> (s? t:f=w382:T9)
        n188 = property on="Ready" class="Bool"("DisabledEnum"=w382) -> ()  [unwired: 2 in, 2 out]
      }
      frame "End PhaseSpace" {
        n189 = Bundle By Name(cluster=w402, "PhaseSpace end?"=TRUE) -> (w401:T6)
      }
      frame "End ATI" {
        n190 = Bundle By Name(cluster=w406, "ATI end?"=TRUE ("PhaseSpace end?")) -> (w405:T6)
      }
      frame "ERROR" {
        # "Error Dialog"
        # "Error is cleared after handling"
        n191 = call <vilib>:"Simple Error Handler.vi"("error in (no error)"=w408) -> ()  [unwired: 4 in, 5 out]
        n192 = call "Error Clear.vi"("error in"=w408) -> ("error in (no error)"=w407:errorcluster)  [unwired: 7 in]
      }
      frame "EXIT" {
        # "Sending exit command to parallel processes"
        n193 = global write "GLOBAL -MAIN.vi" "EXIT"(TRUE ("EXIT")) -> ()
        n194 = Unbundle By Name(w420) -> ("PhaseSpace"=w419:refnum<queue>, "ATI"=w418:refnum<queue>, "trigger task"=w412:refnum<k21>)
        n195 = call <vilib>:"DAQmx Clear Task.vi"("task in"=w412, "error in"=w411) -> ("error out"=w410:errorcluster)  [unwired: 13 in]
        n196 = Enqueue Element(queue=w418, element=cluster{"STATE":T12, "Data":variant} {"STATE"=enum."EXIT", "Data"=variant}, error in (no error)=w410) -> (error out=w421:errorcluster)  [unwired: 1 in, 2 out]
        n197 = Enqueue Element(queue=w419, element=cluster{"STATE":T13, "Data":variant} {"STATE"=enum."EXIT", "Data"=variant}, error in (no error)=w421) -> (error out=w415:errorcluster)  [unwired: 1 in, 2 out]
        n198 = property on="STOP" class="Bool"(error in=w415, "DisabledEnum"=T9."Enabled" ("Disabled")) -> (error out=w414:errorcluster)  [unwired: 1 in, 1 out]
      }
    }
    n199 = call "STTM Q MGR.vi"("QSTATES"=w41, "QRef"=w40, "Error IN"=w48, "FNs"=w42) -> ("Error OUT"=w47:errorcluster)  [unwired: 11 in]
  }
  n200 = Release Queue(queue=w9, force destroy? (F)=TRUE) -> ()  [unwired: 1 in, 3 out]
